vi "Drone Hover.vi"(0 "AT Command Port":refnum<k16>) -> (4 "AT Command Port":refnum<k16>)   [LabVIEW 2011]
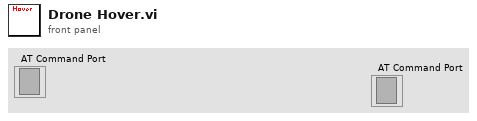
[diagram p1: front panel]
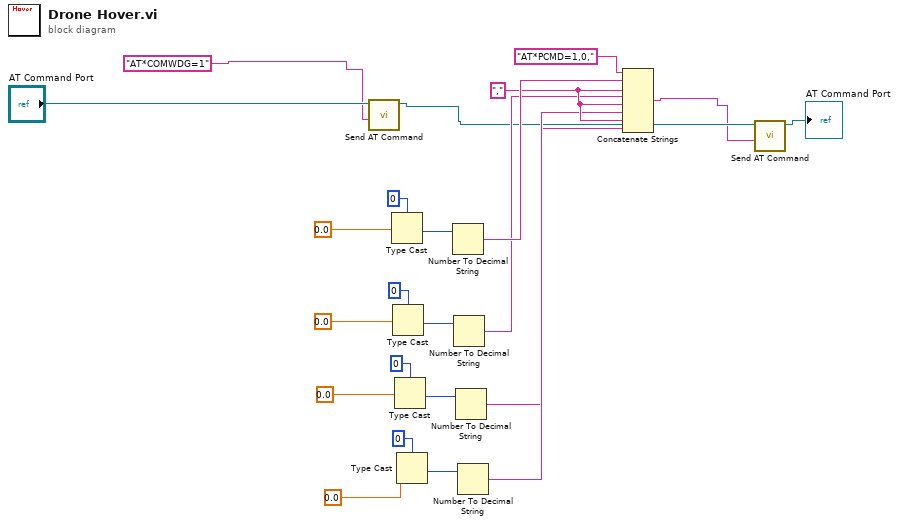
[diagram p0: block diagram]
diagram:
  w17 = ","
  n1 = call "Send AT Command.vi"("AT Command"="AT*COMWDG=1", "AT Command Port"="AT Command Port") -> ("AT Command Port"=w4:refnum<k16>)  [unwired: 9 in]
  n2 = Type Cast(type=u32 0, x=sgl 0.0 ("Roll")) -> (*(type *) &x=w20:u32)
  n3 = Type Cast(type=u32 0, x=sgl 0.0 ("Pitch")) -> (*(type *) &x=w14:u32)
  n4 = Type Cast(type=u32 0, x=sgl 0.0 ("Yaw")) -> (*(type *) &x=w11:u32)
  n5 = Type Cast(type=u32 0, x=sgl 0.0 ("Veritical Speed")) -> (*(type *) &x=w8:u32)
  n6 = Number To Decimal String(number=w20) -> (decimal integer string=w18:string)  [unwired: 1 in]
  n7 = Number To Decimal String(number=w14) -> (decimal integer string=w5:string)  [unwired: 1 in]
  n8 = Number To Decimal String(number=w11) -> (decimal integer string=w6:string)  [unwired: 1 in]
  n9 = Number To Decimal String(number=w8) -> (decimal integer string=w7:string)  [unwired: 1 in]
  n10 = Concatenate Strings("AT*PCMD=1,0,", w18, w17, w5, w17, w7, w17, w6) -> (w1:string)
  n11 = call "Send AT Command.vi"("AT Command"=w1, "AT Command Port"=w4) -> ("AT Command Port"=→"AT Command Port":refnum<k16>)  [unwired: 9 in]
